vi "Network Error.vi"(9 "error in (no error)":errorcluster, 10 "Suppress? (T)":bool=TRUE) -> (1 "error out":errorcluster, 2 "Detected?":bool)   [LabVIEW 2011]
doc: "Checks for standard network communications errors and optionally clears them.\n\n\nVersion 1.0 - 02/13/2013\n\nPhaeron, Inc.\nwww.phaeron.com\ninfo@phaeron.com"
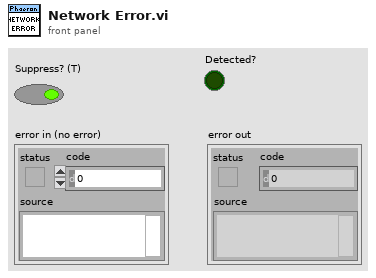
[diagram p1: front panel]
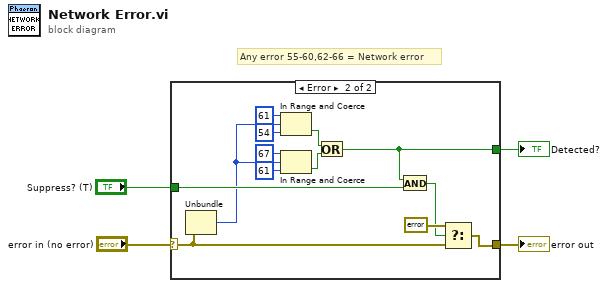
[diagram p0: block diagram]
diagram:
  # "Any error 55-60,62-66 = Network error"
  n1 = case shown="Error" "error in (no error)" {
    selector: "error in (no error)" -> [w5 w18]
    tunnel: [w5 w14] -> w3
    tunnel: "Suppress? (T)" -> [_ w15]
    tunnel: [_ w7] -> w1
    frame No Error {
    }
    frame Error {
      n2 = Unbundle(w18) -> ("code"=w6:i32)  [unwired: 2 out]
      n3 = In Range and Coerce(upper limit=61 ("code"), x=w6, lower limit=54 ("code")) -> (In Range?=w12:bool)  [unwired: 1 out]
      n4 = In Range and Coerce(upper limit=67 ("code"), x=w6, lower limit=61 ("code")) -> (In Range?=w13:bool)  [unwired: 1 out]
      n5 = Or(x=w12, y=w13) -> (x .or. y?=w7:bool)
      n6 = And(x=w7, y=w15) -> (x .and. y?=w16:bool)
      n7 = Select(t=errorcluster {"status"=FALSE, "code"=0, "source"=""}, s=w16, f=w18) -> (s? t:f=w14:errorcluster)
    }
  }
  "error out" <- w3
  "Detected?" <- w1
